vi "CurrentPressure.vi"() -> ()   [LabVIEW 2012]
panel:
  in  "CurrentPressure":dbl
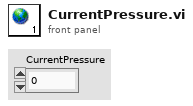
[diagram p1: front panel]
diagram:
